vi "Prepare Insert Command.vi"(8 "Error In (no error)":errorcluster, 10 "Record":variant) -> (0 "Error Out":errorcluster, 2 "Insert SQL Command":string)   [LabVIEW 2023, in "SQLite DB Operator.lvclass"]
uses:
  SQLite DB Operator.lvclass
  <vilib>/JDP Science/JDP Science Common Utilities/Trim Whitespace__JDP.vi
  <userlib>/_OpenG.lib/array/array.llb/Search 1D Array (String)__ogtk.vi
  <userlib>/_OpenG.lib/array/array.llb/Delete Elements from 1D Array (String)__ogtk.vi
  <vilib>/Utility/Data Type/NI_Data Type.lvlib
  <vilib>/drjdpowell/SQLite Library/SQLite.lvlib
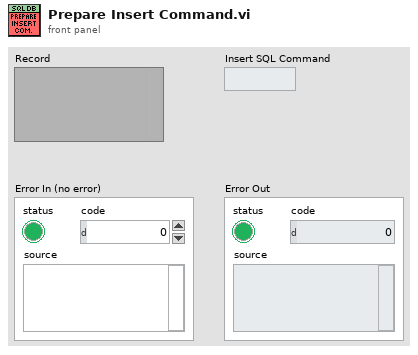
[diagram p1: front panel]
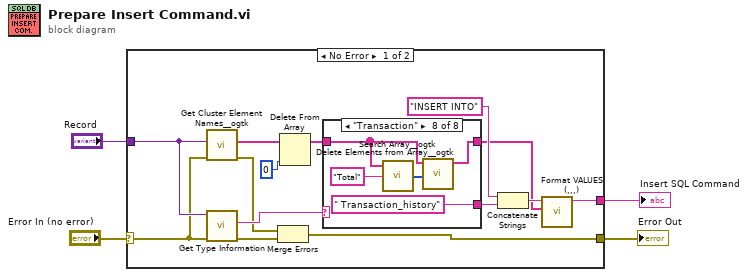
[diagram p0: block diagram]
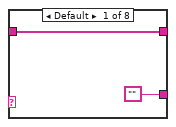
[diagram p2: hidden frame]
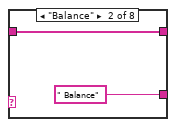
[diagram p3: hidden frame]
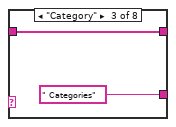
[diagram p4: hidden frame]
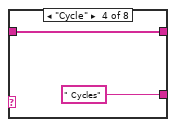
[diagram p5: hidden frame]
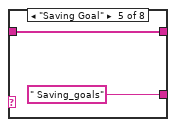
[diagram p6: hidden frame]
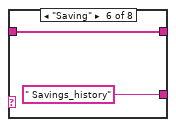
[diagram p7: hidden frame]
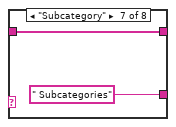
[diagram p8: hidden frame]
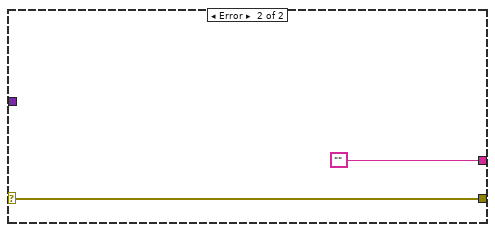
[diagram p9: hidden frame]
diagram:
  n1 = case shown="No Error" "Error In (no error)" {
    selector: "Error In (no error)" -> [w7 w39]
    tunnel: [w16 w39] -> w4
    tunnel: [w13 ""] -> w3
    tunnel: "Record" -> [w8 _]
    frame No Error {
      n2 = call <userlib>:"Get Cluster Element Names__ogtk.vi"("error in (no error)"=w7, "Cluster"=w8) -> ("error out"=w11:errorcluster, "Element Names"=w10:string[])  [unwired: 8 in]
      n3 = call <vilib>:"Get Type Information.vi"("error in (no error)"=w7, "variant"=w8) -> ("error out"=w12:errorcluster, "name"=w18:string)  [unwired: 5 in, 3 out]
      n4 = Merge Errors(w11, w12) -> (w16:errorcluster)
      n5 = Delete From Array(array=w10, index=0) -> (array with subset deleted=w6:string[])  [unwired: 1 in, 1 out]
      n6 = case shown="\"Transaction\"" w18 {
        tunnel: ["" " Balance" ("string") " Categories" ("string") " Cycles" ("string") " Saving_goals" ("string") " Savings_history" ("string") " Subcategories" ("string") " Transaction_history" ("string")] -> w14
        tunnel: w6 -> [w19 w21 w23 w25 w27 w29 w31 w34]
        tunnel: [w19 w21 w23 w25 w27 w29 w31 w33] -> w5
        frame Default {
        }
        frame "Balance" {
        }
        frame "Category" {
        }
        frame "Cycle" {
        }
        frame "Saving Goal" {
        }
        frame "Saving" {
        }
        frame "Subcategory" {
        }
        frame "Transaction" {
          n7 = call-poly <userlib>:"Search Array__ogtk.vi"("Array"=w34, "Element Data"="Total") -> ("Indices of Elements"=w35:i32[])  [unwired: 7 in]
          n8 = call-poly <userlib>:"Delete Elements from Array__ogtk.vi"("indices"=w35, "array"=w34) -> ("array w/ subset deleted"=w33:string[])  [unwired: 8 in, 1 out]
        }
      }
      n9 = Concatenate Strings("INSERT INTO", w14) -> (w15:string)
      n10 = call <vilib>:"Format VALUES (,,,).vi"("Column Names"=w5, "partial SQL"=w15) -> ("SQL"=w13:string)  [unwired: 9 in]
    }
    frame Error {
    }
  }
  "Error Out" <- w4
  "Insert SQL Command" <- w3
